vi "Hardware In - NI 9751-3 (DI Driver).vi"(11 "FPGA Ref":T1) -> ()   [LabVIEW 2015, in "ECS-RT.lvlib"]
uses:
  ECS-RT.lvlib
  Typedefs/FPGA Refs/Generic FPGA Ref.ctl
  <vilib>/Utility/error.llb/Error Cluster From Error Code.vi
  <vilib>/rvi/errors/niLvFpgaAdjustHostInterfaceError.vi
  <vilib>/Powertrain Controls/Device Drivers/Tools/Real-Time/Interp1DTableRT.vi
  <vilib>/rvi/interface/nirviReadWriteControl/nirviReadWriteControl.xnode
  <vilib>/rvi/interface/Simulation/niFpgaSimulationCallBeginRW.vi
  NiFpgaLv.dll
  ECS-Shared.lvlib
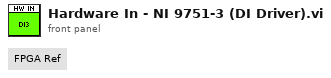
[diagram p1: front panel]
types:
  T1 = typedef "ECS-Shared.lvlib/Generic FPGA Ref.ctl" = refnum<k20>
  T2 = cluster{"ModulePresent":bool, "LVSense":u8, "HVSense":u8, "HVSense2":u8, "TempSense":i8, "Fault1":u8, "Fault2":u8, "OLIntegrator":u32, "HardwareRev":u8, "FirmwareRev":u8}
  T3 = cluster{"FI1OpenCircuit":bool, "FI2OpenCircuit":bool, "FI3OpenCircuit":bool}
  T4 = cluster{"PSCharge":bool, "PSOverLoad":bool, "ShortCircuit":bool, "ModuleTemperature":bool, "HighVoltageDriver":bool, "LowVoltageDriver":bool, "HighVoltageLimit":bool}
  T5 = cluster{"ModulePresent":bool, "Module Temperature (C)":sgl, "Internal High Voltage (V)":sgl, "External High Voltage (V)":sgl, "Battery Voltage (V)":sgl, "Hardware Rev":string, "Firmware Rev":u8}
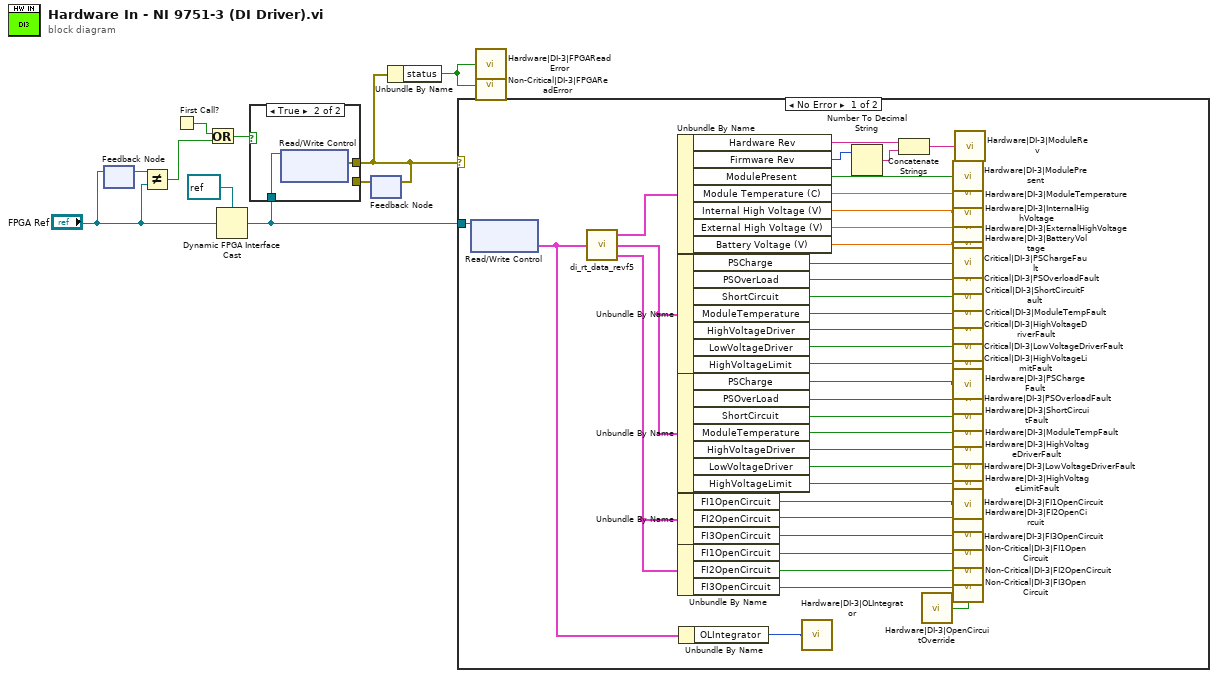
[diagram p0: block diagram]
diagram:
  n1 = feedback #1() -> (w9:T1)  [unwired: 1 in]
  n2 = feedback-in #1("FPGA Ref") -> ()
  n3 = Not Equal?(x=w9, y="FPGA Ref") -> (x != y?=w10:bool)
  n4 = First Call?() -> (First Call?: T/F=w8:bool)
  n5 = Or(x=w8, y=w10) -> (x .or. y?=w7:bool)
  n6 = Dynamic FPGA Interface Cast(Session In=refnum<k20> refnum ("FPGA VI Reference Out"), Type="FPGA Ref") -> (Session Out=w3:refnum<k20>)
  n7 = feedback #2() -> (w6:errorcluster)  [unwired: 1 in]
  n8 = case shown="True" w7 {
    tunnel: [w11 w13] -> w2
    tunnel: w6 -> [w11 _]
    tunnel: w3 -> [_ w12]
    frame False {
    }
    frame True {
      n9 = xnode "Read/Write Control"("FPGA VI Reference In"=w12) -> ("error out"=w13:errorcluster)  [unwired: 1 in, 2 out]
    }
  }
  n10 = feedback-in #2(w2) -> ()
  n11 = Unbundle By Name(w2) -> ("status"=w1:bool)
  n12 = case shown="No Error" w2 {
    tunnel: w3 -> [w14 _]
    frame No Error {
      n13 = xnode "Read/Write Control"("FPGA VI Reference In"=w14) -> ("DI-3.Data"=w15:T2)  [unwired: 1 in, 2 out]
      n14 = call <vilib>:"di_rt_data_revf5.vi"("DIDataFromFPGA"=w15) -> ("Non Critical Faults"=w16:T3, "Critical Faults"=w17:T4, "DIData"=w18:T5)  [unwired: 2 in]
      n15 = Unbundle By Name(w18) -> ("Hardware Rev"=w48:string, "Firmware Rev"=w49:u8, "ModulePresent"=w19:bool, "Module Temperature (C)"=w20:sgl, "Internal High Voltage (V)"=w21:sgl, "External High Voltage (V)"=w22:sgl, "Battery Voltage (V)"=w23:sgl)
      n16 = Unbundle By Name(w17) -> ("PSCharge"=w24:bool, "PSOverLoad"=w25:bool, "ShortCircuit"=w26:bool, "ModuleTemperature"=w27:bool, "HighVoltageDriver"=w28:bool, "LowVoltageDriver"=w29:bool, "HighVoltageLimit"=w30:bool)
      n17 = Unbundle By Name(w17) -> ("PSCharge"=w31:bool, "PSOverLoad"=w32:bool, "ShortCircuit"=w33:bool, "ModuleTemperature"=w34:bool, "HighVoltageDriver"=w35:bool, "LowVoltageDriver"=w36:bool, "HighVoltageLimit"=w37:bool)
      n18 = Unbundle By Name(w16) -> ("FI1OpenCircuit"=w38:bool, "FI2OpenCircuit"=w39:bool, "FI3OpenCircuit"=w40:bool)
      n19 = Unbundle By Name(w16) -> ("FI1OpenCircuit"=w41:bool, "FI2OpenCircuit"=w42:bool, "FI3OpenCircuit"=w43:bool)
      n20 = Unbundle By Name(w15) -> ("OLIntegrator"=w45:u32)
      n21 = call "Hardware|DI-3|OLIntegrator"("Value"=w45) -> ()
      n22 = Number To Decimal String(number=w49) -> (decimal integer string=w47:string)  [unwired: 1 in]
      n23 = Concatenate Strings(w48, w47) -> (w46:string)
      n24 = call "Hardware|DI-3|OpenCircuitOverride"() -> ("Value"=w44:bool)
      n25 = call "Hardware|DI-3|ModulePresent"("Value"=w19) -> ()
      n26 = call "Hardware|DI-3|ModuleTemperature"("Value"=w20) -> ()
      n27 = call "Hardware|DI-3|InternalHighVoltage"("Value"=w21) -> ()
      n28 = call "Hardware|DI-3|ExternalHighVoltage"("Value"=w22) -> ()
      n29 = call "Hardware|DI-3|BatteryVoltage"("Value"=w23) -> ()
      n30 = call "Critical|DI-3|PSChargeFault"("Fault"=w24) -> ()  [unwired: 2 in]
      n31 = call "Critical|DI-3|PSOverloadFault"("Fault"=w25) -> ()  [unwired: 2 in]
      n32 = call "Critical|DI-3|ShortCircuitFault"("Fault"=w26) -> ()  [unwired: 2 in]
      n33 = call "Critical|DI-3|ModuleTempFault"("Fault"=w27) -> ()  [unwired: 2 in]
      n34 = call "Critical|DI-3|HighVoltageDriverFault"("Fault"=w28) -> ()  [unwired: 2 in]
      n35 = call "Critical|DI-3|LowVoltageDriverFault"("Fault"=w29) -> ()  [unwired: 2 in]
      n36 = call "Critical|DI-3|HighVoltageLimitFault"("Fault"=w30) -> ()  [unwired: 2 in]
      n37 = call "Hardware|DI-3|PSChargeFault"("Value"=w31) -> ()
      n38 = call "Hardware|DI-3|PSOverloadFault"("Value"=w32) -> ()
      n39 = call "Hardware|DI-3|ShortCircuitFault"("Value"=w33) -> ()
      n40 = call "Hardware|DI-3|ModuleTempFault"("Value"=w34) -> ()
      n41 = call "Hardware|DI-3|HighVoltageDriverFault"("Value"=w35) -> ()
      n42 = call "Hardware|DI-3|LowVoltageDriverFault"("Value"=w36) -> ()
      n43 = call "Hardware|DI-3|HighVoltageLimitFault"("Value"=w37) -> ()
      n44 = call "Hardware|DI-3|FI1OpenCircuit"("Value"=w38) -> ()
      n45 = call "Hardware|DI-3|FI2OpenCircuit"("Value"=w39) -> ()
      n46 = call "Hardware|DI-3|FI3OpenCircuit"("Value"=w40) -> ()
      n47 = call "Non-Critical|DI-3|FI1OpenCircuit"("Fault"=w41, "Override (F)"=w44) -> ()  [unwired: 1 in]
      n48 = call "Non-Critical|DI-3|FI2OpenCircuit"("Fault"=w42, "Override (F)"=w44) -> ()  [unwired: 1 in]
      n49 = call "Non-Critical|DI-3|FI3OpenCircuit"("Fault"=w43, "Override (F)"=w44) -> ()  [unwired: 1 in]
      n50 = call "Hardware|DI-3|ModuleRev"("Value"=w46) -> ()
    }
    frame Error {
    }
  }
  n51 = call "Hardware|DI-3|FPGAReadError"("Value"=w1) -> ()
  n52 = call "Non-Critical|DI-3|FPGAReadError"("Fault"=w1) -> ()  [unwired: 2 in]
